vi "Start Move.vi"(8 "error in (no error)":errorcluster, 11 "SwipeMenu in":refnum<class "SwipeMenu.lvclass">) -> (0 "error out":errorcluster, 2 "Mouse Down?":bool, 3 "SwipeMenu out":refnum<class "SwipeMenu.lvclass">)   [LabVIEW 2019, in "SwipeMenu.lvclass"]
uses:
  SwipeMenu.lvclass
  SwipeMenu.lvclass/SwipeMenu.ctl
  <vilib>/Utility/inputDevices.llb/mouseAcquire.vi
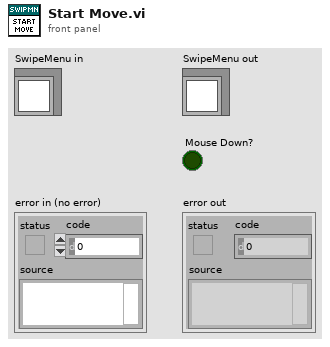
[diagram p1: front panel]
types:
  T1 = typedef "LVPointTypeDef.ctl" = cluster{"Horizontal":i16, "Vertical":i16}
  T2 = cluster{"Horizontal":i32, "Vertical":i32, "Scrolling":i32}
  T3 = cluster{"button 1":bool, "button 2":bool, "button 3":bool, "button 4":bool}
  T4 = enum16{"Idle", "Mouse Nav", "Slowdown", "Button Nav"}
  T5 = typedef "SwipeMenu.lvclass/State Data.ctl" = cluster{"State":enum16{"Idle", "Mouse Nav", "Slowdown", "Button Nav"}, "Timeout":i32, "Time":timestamp, "Position":i32, "Scroll Position":i16, "Rate":dbl, "Direction":enum16{"Left", "Right"}}
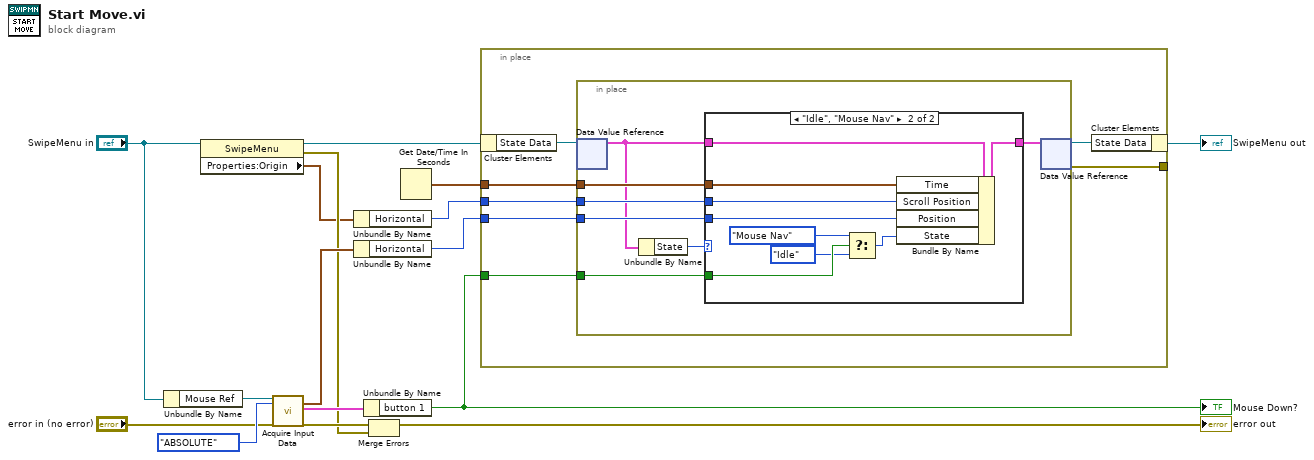
[diagram p0: block diagram]
diagram:
  n1 = Unbundle By Name("SwipeMenu in") -> ("Mouse Ref"=w15:refnum<k1>)
  n2 = property class="SwipeMenu"(reference="SwipeMenu in") -> (reference out=w4:refnum<class "SwipeMenu.lvclass">, error out=w3:errorcluster, "Properties:Origin"=w2:T1)  [unwired: 1 in]
  n3 = call-poly <vilib>:"Acquire Input Data.vi"("device ID"=w15, "key mode"=enum16{"RELATIVE", "ABSOLUTE"}."ABSOLUTE", "error in (no error)"="error in (no error)") -> ("axis info"=w11:T2, "button info"=w12:T3, "error out"=w13:errorcluster)  [unwired: 13 in, 1 out]
  n4 = Unbundle By Name(w2) -> ("Horizontal"=w8:i16)
  n5 = Unbundle By Name(w11) -> ("Horizontal"=w7:i32)
  n6 = Unbundle By Name(w12) -> ("button 1"=w1:bool)
  "Mouse Down?" <- w1
  n7 = Merge Errors(w13, w3) -> (→"error out":errorcluster)
  n8 = Get Date/Time In Seconds() -> (seconds since 1Jan1904=w9:timestamp)
  n9 = in-place {
    in-place-border: w9 -> [w21]
    in-place-border: [w20] -> _
    in-place-border: w8 -> [w19]
    in-place-border: w7 -> [w18]
    in-place-border: w1 -> [w17]
    n10 = in-place-cluster #1(w4) -> ("State Data"=w23:refnum<data-value>)
    n11 = in-place {
      in-place-border: w21 -> [w29]
      in-place-border: w19 -> [w27]
      in-place-border: w18 -> [w28]
      in-place-border: w17 -> [w26]
      n12 = in-place-dvr #2(w23) -> (w25:T5)  [unwired: 1 out]
      n13 = Unbundle By Name(w25) -> ("State"=w24:T4)
      n14 = case shown="\"Idle\", \"Mouse Nav\"" w24 {
        tunnel: [w31 w40] -> w30
        tunnel: w29 -> [_ w39]
        tunnel: w28 -> [_ w38]
        tunnel: w27 -> [_ w37]
        tunnel: w26 -> [_ w36]
        tunnel: w25 -> [w31 w33]
        frame Default {
        }
        frame "Idle", "Mouse Nav" {
          n15 = Select(t=T4."Mouse Nav" ("State"), s=w36, f=T4."Idle") -> (s? t:f=w32:T4)
          n16 = Bundle By Name(cluster=w33, "Time"=w39, "Scroll Position"=w37, "Position"=w38, "State"=w32) -> (w40:T5)
        }
      }
      n17 = in-place-dvr #2(w30) -> (w22:refnum<data-value>, w20:errorcluster)
    }
    n18 = in-place-cluster #1("State Data"=w22) -> (→"SwipeMenu out":refnum<class "SwipeMenu.lvclass">)
  }
